vi "Amp_PS_getd.vi"(5 "Amp PS address":refnum<visa-resource-name>, 6 "delay before read (ms)":u32=500, 7 "error in (no error)":errorcluster) -> (0 "voltage, V":dbl, 1 "current, A":dbl, 2 "status":bool, 3 "output cluster":T1, 4 "mode":i32(ring)=-1 items=["CV", "CC"])   [LabVIEW 2010]
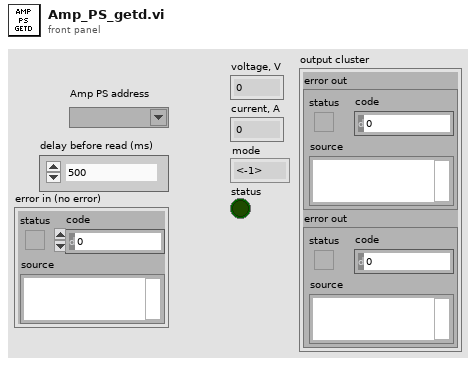
[diagram p1: front panel]
types:
  T1 = cluster{"error out":errorcluster, "error out":errorcluster}
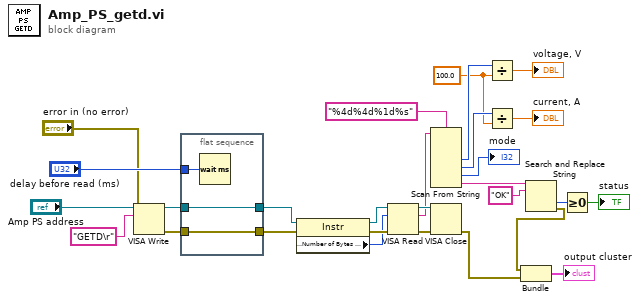
[diagram p0: block diagram]
diagram:
  w10 = 100.0 ("y")
  n1 = VISA Write(VISA resource name="Amp PS address", write buffer="GETD\r", error in (no error)="error in (no error)") -> (VISA resource name out=w24:refnum<visa-resource-name>, error out=w26:errorcluster)  [unwired: 1 out]
  n2 = flat-sequence {
    tunnel: w26 -> [w30]
    tunnel: [w30] -> w25
    tunnel: w24 -> [w29]
    tunnel: [w29] -> w23
    tunnel: "delay before read (ms)" -> [w31]
    frame #0 {
      n3 = Wait (ms)(milliseconds to wait=w31) -> ()  [unwired: 1 out]
    }
  }
  n4 = property class="Instr"(reference=w23, error in=w25) -> (reference out=w22:refnum<visa-resource-name>, error out=w21:errorcluster, "Serial Settings:Number of Bytes at Serial Port"=w20:u32)
  n5 = VISA Read(VISA resource name=w22, byte count=w20, error in (no error)=w21) -> (VISA resource name out=w27:refnum<visa-resource-name>, read buffer=w13:string, error out=w28:errorcluster)  [unwired: 1 out]
  n6 = Scan From String(format string="%4d%4d%1d%s", input string=w13) -> (output 1=w12:i32, output 2=w11:i32, output 3=→"mode":i32, output 4=w6:string)  [unwired: 6 in, 3 out]
  n7 = VISA Close(VISA resource name=w27, error in (no error)=w28) -> (error out=w2:errorcluster)
  n8 = Divide(x=w12, y=w10) -> (x/y=→"voltage, V":dbl)
  n9 = Divide(x=w11, y=w10) -> (x/y=→"current, A":dbl)
  n10 = Search and Replace String(input string=w6, search string="OK" ("true string")) -> (offset past replacement=w15:i32, error out=w3:errorcluster)  [unwired: 6 in, 2 out]
  n11 = Bundle("error out"=w3, "error out"=w2) -> (→"output cluster":T1)  [unwired: 1 in]
  n12 = Greater Or Equal To 0?(x=w15) -> (x >= 0?=→"status":bool)
